vi "mhk_Cont Acq&Chart Samples-SW Timed.vi"() -> ()   [LabVIEW 2010]
doc: "I. Description:\nThis example demonstrates how to continuously acquire data (waveform) using software timing (rate is governed by while loop iteration interval).\n\nII. Instructions for Running:\n1. Select the physical channel to correspond to where your signal is input on the DAQ device.\n2. Enter the minimum and maximum voltage ranges.\nNote: For better accuracy try to match the input range to the expected voltage level of the measured signal.\n\nIII. Block Diagram Steps:\n1. Create an analog input voltage channel.\n2. Call the Start VI to start the task.\n3. Read the waveform data in a loop until the user hits the stop\nbutton or an error occurs.\n4. Call the Clear Task VI to clear the Task.\n5. Use the popup dialog box to display an error if any.\n\nIV. I/O Connections Overview:\nMake sure your signal input terminal matches the Physical Channel I/O control."
uses:
  <vilib>/Utility/error.llb/DialogType.ctl
  <vilib>/DAQmx/read.llb/DAQmx Read (Analog 1D Wfm NChan 1Samp).vi
  <vilib>/DAQmx/create/channels.llb/DAQmx Create Channel (AI-Voltage-Basic).vi
  <vilib>/daqmx/miscellaneous.llb/DAQmx Fill In Error Info.vi
panel:
  in  "Software Loop Time (ms)":u32=250
  in  "Physical Channel":tag="Dev1/ai0"
  in  "Minimum Value":dbl=-10.0 format="%0.2f"
  in  "Maximum Value":dbl=10.0 format="%0.2f"
  in  "stop":bool
  out "Measurement":waveform(dbl)[](graph)=[{"t0"=timestamp(3130167226.168554 s since 1904-01-01), "dt"=1.0, "Y"=[0.2587890625], "attributes"=variant("NI_ChannelName"=variant(string "Dev1/ai0"), "NI_UnitDescription"=variant(string "Volts"))}]
  # "For instructions, select Help>>Show Context Help"
  # "Timing Parameters"
  # "Channel Parameters"
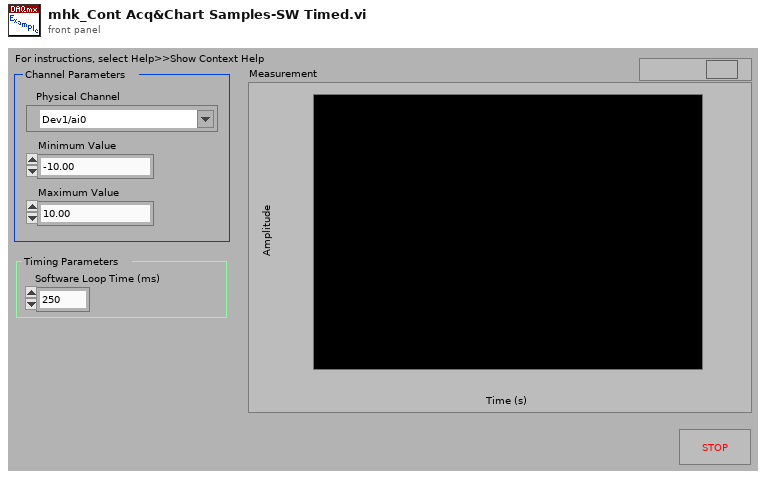
[diagram p1: front panel]
types:
  T1 = typedef "DialogType.ctl" = u16
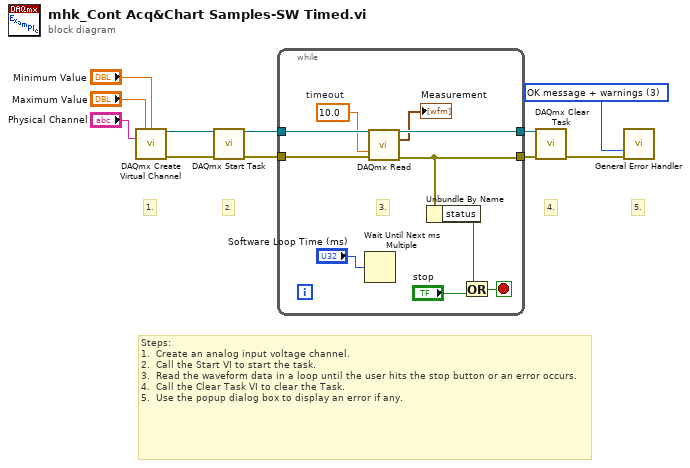
[diagram p0: block diagram]
diagram:
  w1 = T1 3 items=["no dialog", "OK message", "continue or stop message", "OK message + warnings", "continue/stop + warnings"] ("type of dialog (OK msg:1)")
  # "5."
  # "2."
  # "Steps: \n1.  Create an analog input voltage channel.\n2.  Call the Start VI to start the task.\n3.  Read the waveform data in a loop until the user hits the stop button or an error occurs.\n4.  Call the Clear Task VI to clear the Task.\n5.  Use the popup dialog box to display an error if any."
  # "4."
  # "1."
  n1 = call-poly <vilib>:"DAQmx Create Virtual Channel.vi"("maximum value"="Maximum Value", "minimum value"="Minimum Value", "physical channels"="Physical Channel") -> ("task out"=w3:refnum<k21>, "error out"=w2:errorcluster)  [unwired: 11 in]
  n2 = call <vilib>:"DAQmx Start Task.vi"("task/channels in"=w3, "error in"=w2) -> ("task out"=w6:refnum<k21>, "error out"=w9:errorcluster)  [unwired: 12 in]
  n3 = while {
    tunnel: w9 -> [w21]
    tunnel: [w17] -> w8
    tunnel: w6 -> [w16]
    tunnel: [w15] -> w5
    stop <- w20 stop-if-true
    w13 = 10.0  # timeout
    # "3."
    n4 = Wait Until Next ms Multiple(millisecond multiple="Software Loop Time (ms)") -> ()  [unwired: 1 out]
    n5 = call-poly <vilib>:"DAQmx Read.vi"("task/channels in"=w16, "timeout"=w13, "error in"=w21) -> ("task out"=w15:refnum<k21>, "data"=→"Measurement":waveform(dbl)[], "error out"=w17:errorcluster)  [unwired: 10 in]
    n6 = Unbundle By Name(w17) -> ("status"=w18:bool)
    n7 = Or(x=w18, y="stop") -> (x .or. y?=w20:bool)
  }
  n8 = call <vilib>:"DAQmx Clear Task.vi"("task in"=w5, "error in"=w8) -> ("error out"=w7:errorcluster)  [unwired: 13 in]
  n9 = call <vilib>:"General Error Handler.vi"("type of dialog (OK msg:1)"=w1, "error in (no error)"=w7) -> ()  [unwired: 9 in, 5 out]
